vi "STATE_MACHINE_SIMPLE_PICKUPp.vi"() -> ()   [LabVIEW 2018]
uses:
  STATE_MACHINE_SIMPLE_PICKUP_TYPEDEF.ctl
  Underlying VI's/I2C Master VI/I2C_MASTER_WRITE.ctl
panel:
  out "error out":errorcluster
  out "State":T1
  out "cluster":T2
  in  "Start task":bool
  in  "Steppers homed?":bool
  in  "stop":bool
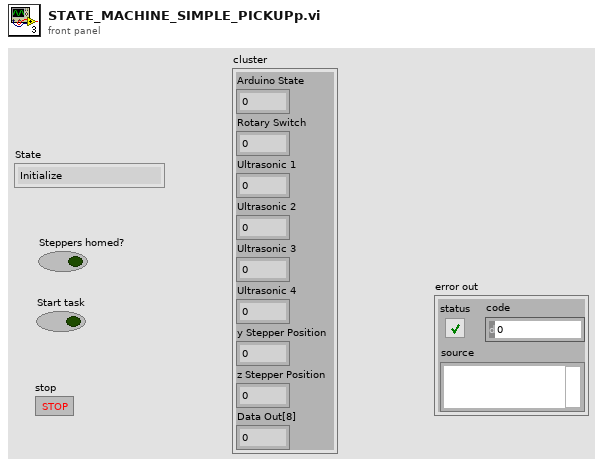
[diagram p1: front panel]
types:
  T1 = typedef "STATE_MACHINE_SIMPLE_PICKUP_TYPEDEF.ctl" = enum16{"Initialize", "Check steppers home", "Idle", "Move y stepper front", "Move z stepper down", "Grab", "Grab Delay", "Release", "Release Delay"}
  T2 = cluster{"Arduino State":u8, "Rotary Switch":u8, "Ultrasonic 1":u8, "Ultrasonic 2":u8, "Ultrasonic 3":u8, "Ultrasonic 4":u8, "y Stepper Position":u8, "z Stepper Position":u8, "Data Out[8]":u8}
  T3 = typedef "I2C_MASTER_WRITE.ctl" = enum16{"Ultrasonic sensors", "Stepper origin", "zStepper 13.3k", "zStepper 13k", "zStepper 12k", "zStepper 11k", "zStepper 10k", "zStepper 9k", "zStepper 8k", "zStepper 7k", "zStepper 6k", "zStepper 5k", "zStepper 4k", "zStepper 3k", "zStepper 2k", "zStepper 1k", "zStepper 900", "zStepper 800", "zStepper 700", "zStepper 600", "zStepper 500", "zStepper 400", "zStepper 300", "zStepper 200", "zStepper 100", "zStepper 0", "yStepper 4.7k", "yStepper 4.6k", "yStepper 4.5k", "yStepper 4.4k", "yStepper 4.3k", "yStepper 4.2k", "yStepper 4.1k", "yStepper 4k", "yStepper 3.9k", "yStepper 3.8k", "yStepper 3.7k", "yStepper 3.6k", "yStepper 3.5k", "yStepper 3.4k", "yStepper 3.3k", "yStepper 3.2k", "yStepper 3.1k", "yStepper 3k", "yStepper 2.9k", "yStepper 2.8k", "yStepper 2.7k", "yStepper 2.6k", "yStepper 2.5k", "yStepper 2.4k", "yStepper 2.3k", "yStepper 2.2k", "yStepper 2.1k", "yStepper 2k", "yStepper 1.9k", "yStepper 1.8k", "yStepper 1.7k", "yStepper 1.6k", "yStepper 1.5k", "yStepper 1.4k", "yStepper 1.3k", "yStepper 1.2k", "yStepper 1.1k", "yStepper 1k", "yStepper 900", "yStepper 800", "yStepper 700", "ySteppre 600", "yStepper 500", "yStepper 400", "yStepper 300", "yStepper 200", "yStepper 100", "yStepper 0", "Open claw", "Close claw", "Last State"}
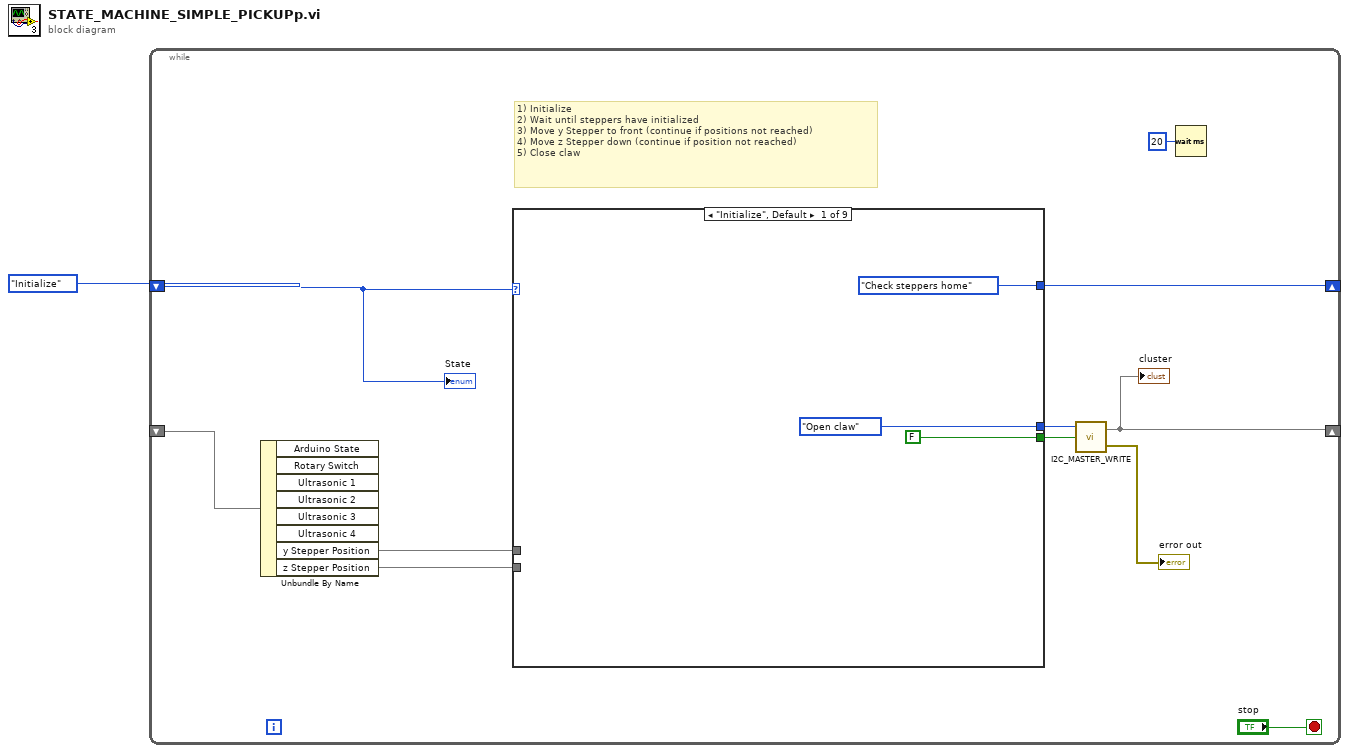
[diagram p0: block diagram]
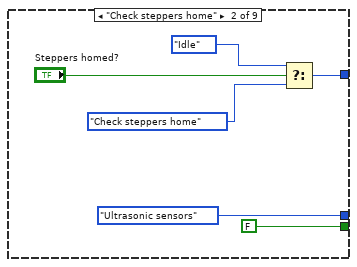
[diagram p2: hidden frame]
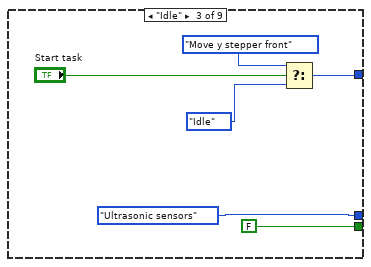
[diagram p3: hidden frame]
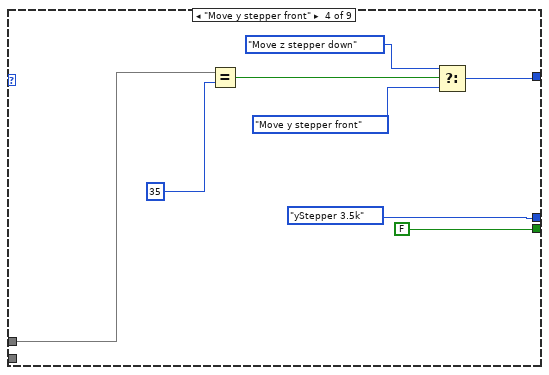
[diagram p4: hidden frame]
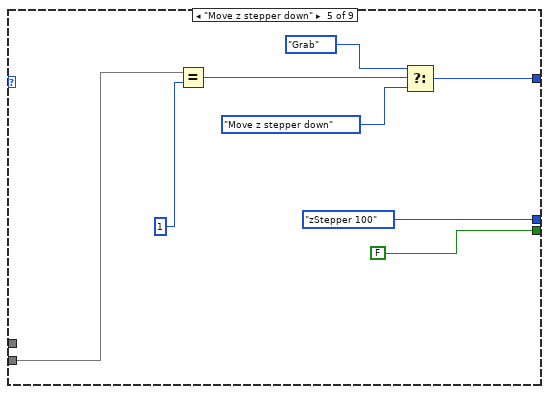
[diagram p5: hidden frame]
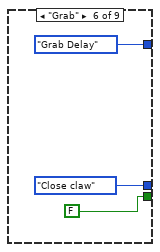
[diagram p6: hidden frame]
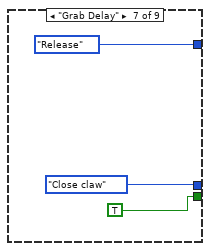
[diagram p7: hidden frame]
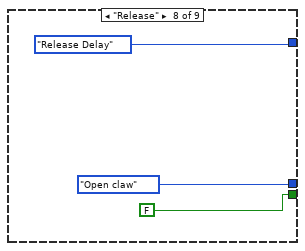
[diagram p8: hidden frame]
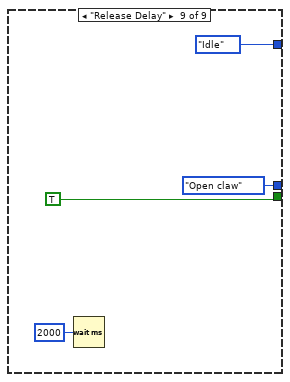
[diagram p9: hidden frame]
diagram:
  n1 = while {
    shift-right: [w9] -> _
    shift-left: STATE_MACHINE_SIMPLE_PICKUP_TYPEDEF."Initialize" -> [w11]
    shift-right: [w6] -> _
    shift-left: _ -> [w5]
    stop <- "stop" stop-if-true
    # "1) Initialize\n2) Wait until steppers have initialized\n3) Move y Stepper to front (continue if positions not reached)\n4) Move z Stepper down (continue if position not reached)\n5) Close claw"
    n2 = Unbundle By Name(w5) -> ("y Stepper Position"=w4, "z Stepper Position"=w3)  [unwired: 6 out]
    n3 = case shown="\"Initialize\", Default" w11 {
      tunnel: [STATE_MACHINE_SIMPLE_PICKUP_TYPEDEF."Check steppers home" w20 w24 w33 w38 STATE_MACHINE_SIMPLE_PICKUP_TYPEDEF."Grab Delay" STATE_MACHINE_SIMPLE_PICKUP_TYPEDEF."Release" STATE_MACHINE_SIMPLE_PICKUP_TYPEDEF."Release Delay" STATE_MACHINE_SIMPLE_PICKUP_TYPEDEF."Idle"] -> w9
      tunnel: [I2C_MASTER_WRITE."Open claw" ("Mode") I2C_MASTER_WRITE."Ultrasonic sensors" ("Mode") I2C_MASTER_WRITE."Ultrasonic sensors" ("Mode") I2C_MASTER_WRITE."yStepper 3.5k" ("Mode") I2C_MASTER_WRITE."zStepper 100" ("Mode") I2C_MASTER_WRITE."Close claw" ("Mode") I2C_MASTER_WRITE."Close claw" ("Mode") I2C_MASTER_WRITE."Open claw" ("Mode") I2C_MASTER_WRITE."Open claw" ("Mode")] -> w8
      tunnel: [FALSE ("Latch") FALSE ("Latch") FALSE ("Latch") FALSE ("Latch") FALSE ("Latch") FALSE ("Latch") TRUE ("Latch") FALSE ("Latch") TRUE ("Latch")] -> w7
      tunnel: w4 -> [_ _ _ w29 _ _ _ _ _]
      tunnel: w3 -> [_ _ _ _ w37 _ _ _ _]
      frame "Initialize", Default {
      }
      frame "Check steppers home" {
        n4 = Select(t=STATE_MACHINE_SIMPLE_PICKUP_TYPEDEF."Idle", s="Steppers homed?", f=STATE_MACHINE_SIMPLE_PICKUP_TYPEDEF."Check steppers home") -> (s? t:f=w20:T1)
      }
      frame "Idle" {
        n5 = Select(t=STATE_MACHINE_SIMPLE_PICKUP_TYPEDEF."Move y stepper front", s="Start task", f=STATE_MACHINE_SIMPLE_PICKUP_TYPEDEF."Idle") -> (s? t:f=w24:T1)
      }
      frame "Move y stepper front" {
        n6 = Equal?(x=w29, y=u8 35) -> (x = y?=w30:bool)
        n7 = Select(t=STATE_MACHINE_SIMPLE_PICKUP_TYPEDEF."Move z stepper down", s=w30, f=STATE_MACHINE_SIMPLE_PICKUP_TYPEDEF."Move y stepper front") -> (s? t:f=w33:T1)
      }
      frame "Move z stepper down" {
        n8 = Equal?(x=w37, y=u8 1) -> (x = y?=w41:bool)
        n9 = Select(t=STATE_MACHINE_SIMPLE_PICKUP_TYPEDEF."Grab", s=w41, f=STATE_MACHINE_SIMPLE_PICKUP_TYPEDEF."Move z stepper down") -> (s? t:f=w38:T1)
      }
      frame "Grab" {
      }
      frame "Grab Delay" {
      }
      frame "Release" {
      }
      frame "Release Delay" {
        n10 = Wait (ms)(milliseconds to wait=u32 2000) -> ()  [unwired: 1 out]
      }
    }
    n11 = call "I2C_MASTER_WRITE.vi"("Latch"=w7, "Mode"=w8) -> ("error out"=→"error out":errorcluster, 1:w6)  [unwired: 1 in]
    "cluster" <- w6
    n12 = Wait (ms)(milliseconds to wait=u32 20) -> ()  [unwired: 1 out]
    "State" <- w11
  }
